vi "log flow rates.vi"(6 "odor 2 setpoint":dbl, 7 "numPidReadings":i32=83, 8 "error in":errorcluster, 9 "odor 1 setpoint":dbl, 10 "air flow set point":dbl, 11 "daqmx tasks":T2) -> (0 "error out":errorcluster, 2 "flow rates":T1 {"pid reading" format="%0.2f"})   [LabVIEW 2013]
uses:
  <vilib>/DAQmx/read.llb/DAQmx Read (Analog DBL 1Chan 1Samp).vi
  <vilib>/DAQmx/read.llb/DAQmx Read (Analog 1D DBL 1Chan NSamp).vi
  <vilib>/Analysis/baseanly.llb/Mean (DBL).vi
  <vilib>/DAQmx/miscellaneous.llb/DAQmx Fill In Error Info.vi
  <vilib>/Analysis/NI_AALBase.lvlib
panel:
  in  "co2 setpoint":dbl
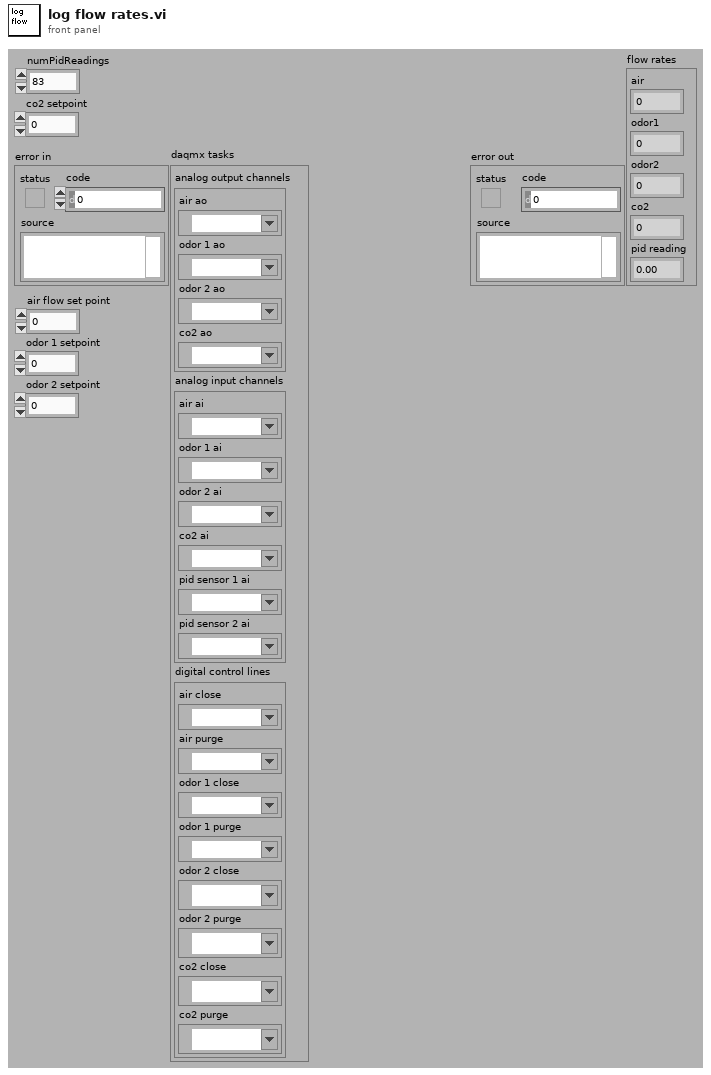
[diagram p1: front panel]
types:
  T1 = cluster{"air":dbl, "odor1":dbl, "odor2":dbl, "co2":dbl, "pid reading":dbl}
  T2 = cluster{"analog output channels":cluster{"air ao":refnum<k21>, "odor 1 ao":refnum<k21>, "odor 2 ao":refnum<k21>, "co2 ao":refnum<k21>}, "analog input channels":cluster{"air ai":refnum<k21>, "odor 1 ai":refnum<k21>, "odor 2 ai":refnum<k21>, "co2 ai":refnum<k21>, "pid sensor 1 ai":refnum<k21>, "pid sensor 2 ai":refnum<k21>}, "digital control lines":cluster{"air close":refnum<k21>, "air purge":refnum<k21>, "odor 1 close":refnum<k21>, "odor 1 purge":refnum<k21>, "odor 2 close":refnum<k21>, "odor 2 purge":refnum<k21>, "co2 close":refnum<k21>, "co2 purge":refnum<k21>}}
  T3 = enum16{"Reset Table", "Get Values", "Add Value", "Get Table", "Get Spreadsheet", "set stack writer"}
  T4 = cluster{"data":dbl, "data":dbl, "data":dbl, "data":dbl, "mean":dbl}
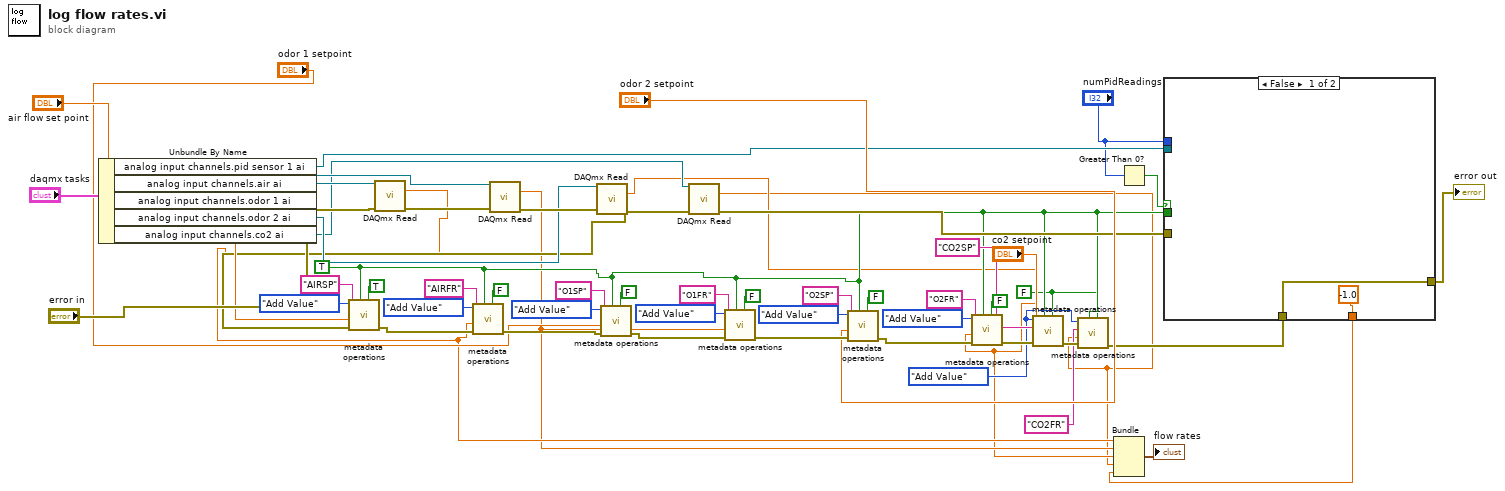
[diagram p0: block diagram]
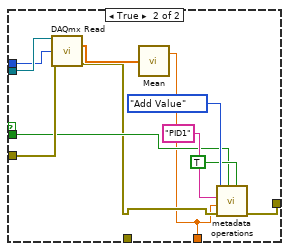
[diagram p2: hidden frame]
diagram:
  w13 = T3."Add Value" ("Operation")
  w11 = FALSE ("add time?")
  w12 = TRUE ("add to stack writer")
  n1 = Unbundle By Name("daqmx tasks") -> ("analog input channels.pid sensor 1 ai"=w22:refnum<k21>, "analog input channels.air ai"=w53:refnum<k21>, "analog input channels.odor 1 ai"=w51:refnum<k21>, "analog input channels.odor 2 ai"=w49:refnum<k21>, "analog input channels.co2 ai"=w18:refnum<k21>)
  n2 = call-poly <vilib>:"DAQmx Read.vi"("task/channels in"=w53, "error in"="error in") -> ("data"=w6:dbl, "error out"=w52:errorcluster)  [unwired: 11 in, 1 out]
  n3 = call-poly <vilib>:"DAQmx Read.vi"("task/channels in"=w51, "error in"=w52) -> ("data"=w5:dbl, "error out"=w50:errorcluster)  [unwired: 11 in, 1 out]
  n4 = call-poly <vilib>:"DAQmx Read.vi"("task/channels in"=w49, "error in"=w50) -> ("data"=w4:dbl, "error out"=w20:errorcluster)  [unwired: 11 in, 1 out]
  n5 = call "metadata operations.vi"("add time?"=TRUE, "add to stack writer"=w12, "error in (no error)"=w20, "value"="air flow set point", "key"="AIRSP", "Operation"=T3."Add Value") -> ("error out"=w42:errorcluster)  [unwired: 2 in, 3 out]
  n6 = call "metadata operations.vi"("add time?"=FALSE, "add to stack writer"=w12, "error in (no error)"=w42, "value"=w6, "key"="AIRFR", "Operation"=T3."Add Value") -> ("error out"=w35:errorcluster)  [unwired: 2 in, 3 out]
  n7 = call "metadata operations.vi"("add time?"=FALSE, "add to stack writer"=w12, "error in (no error)"=w35, "value"="odor 1 setpoint", "key"="O1SP", "Operation"=T3."Add Value") -> ("error out"=w36:errorcluster)  [unwired: 2 in, 3 out]
  n8 = call-poly <vilib>:"DAQmx Read.vi"("task/channels in"=w18, "error in"=w20) -> ("data"=w3:dbl, "error out"=w19:errorcluster)  [unwired: 11 in, 1 out]
  n9 = call "metadata operations.vi"("add time?"=FALSE, "add to stack writer"=w12, "error in (no error)"=w36, "value"=w5, "key"="O1FR", "Operation"=T3."Add Value") -> ("error out"=w28:errorcluster)  [unwired: 2 in, 3 out]
  n10 = call "metadata operations.vi"("add time?"=FALSE, "add to stack writer"=w12, "error in (no error)"=w28, "value"="odor 2 setpoint", "key"="O2SP", "Operation"=T3."Add Value") -> ("error out"=w29:errorcluster)  [unwired: 2 in, 3 out]
  n11 = call "metadata operations.vi"("add time?"=FALSE, "add to stack writer"=w12, "error in (no error)"=w29, "value"=w4, "key"="O2FR", "Operation"=T3."Add Value") -> ("error out"=w17:errorcluster)  [unwired: 2 in, 3 out]
  n12 = call "metadata operations.vi"("add time?"=w11, "add to stack writer"=w12, "error in (no error)"=w17, "value"="co2 setpoint", "key"="CO2SP", "Operation"=w13) -> ("error out"=w14:errorcluster)  [unwired: 2 in, 3 out]
  n13 = call "metadata operations.vi"("add time?"=w11, "add to stack writer"=w12, "error in (no error)"=w14, "value"=w3, "key"="CO2FR", "Operation"=w13) -> ("error out"=w7:errorcluster)  [unwired: 2 in, 3 out]
  n14 = Greater Than 0?(x="numPidReadings") -> (x > 0?=w8:bool)
  n15 = case shown="False" w8 {
    tunnel: w22 -> [_ w68]
    tunnel: "numPidReadings" -> [_ w66]
    tunnel: [w57 w65] -> w21
    tunnel: w19 -> [_ w61]
    tunnel: w12 -> [_ w60]
    tunnel: w7 -> [w57 _]
    tunnel: [-1.0 ("mean") w58] -> w1
    frame False {
    }
    frame True {
      n16 = call-poly <vilib>:"DAQmx Read.vi"("task/channels in"=w68, "number of samples per channel"=w66, "error in"=w61) -> ("data"=w67:dbl[], "error out"=w59:errorcluster)  [unwired: 10 in, 1 out]
      n17 = call-poly <vilib>:"Mean.vi"("X"=w67) -> ("mean"=w58:dbl)  [unwired: 1 out]
      n18 = call "metadata operations.vi"("add time?"=TRUE, "add to stack writer"=w60, "error in (no error)"=w59, "value"=w58, "key"="PID1", "Operation"=T3."Add Value") -> ("error out"=w65:errorcluster)  [unwired: 2 in, 3 out]
    }
  }
  "error out" <- w21
  n19 = Bundle("data"=w6, "data"=w5, "data"=w4, "data"=w3, "mean"=w1) -> (→"flow rates":T4)  [unwired: 1 in]
